vi "Setpoint.vi"(8 "error in (no error)":errorcluster, 10 "Setpoint [A]":dbl format="%.5f", 11 "PS Driver AMI4xx.lvlib:PS Driver AMI4xx.lvclass in":refnum<class "PS Driver AMI4xx.lvclass">) -> (0 "error out":errorcluster, 2 "Setpoint out (A)":dbl, 3 "PS Driver AMI4xx.lvlib:PS Driver AMI4xx.lvclass out":refnum<class "PS Driver AMI4xx.lvclass">)   [LabVIEW 2025, in "PS Driver.lvlib" / "PS Driver AMI4xx.lvclass"]
doc: "Author: Scott Hannahs <sth@magnet.fsu.edu>\n\nThis software is licensed for use under the “MIT License\"\nCopyright (c) 2025 Scott Hannahs, sth@sth@magnet.sthnet.net\n\nPermission is hereby granted, free of charge, to any person obtaining a copy of this software and associated documentation files (the \"Software\"), to deal in the Software without restriction, including without limitation the rights to use, copy, modify, merge, publish, distribute, sublicense, and/or sell copies of the Software, and to permit persons to whom the Software is furnished to do so, subject to the following conditions: The above copyright notice and this permission notice shall be included in all copies or substantial portions of the Software.\n\nTHE SOFTWARE IS PROVIDED \"AS IS\", WITHOUT WARRANTY OF ANY KIND, EXPRESS OR IMPLIED, INCLUDING BUT NOT LIMITED TO THE WARRANTIES OF MERCHANTABILITY, FITNESS FOR A PARTICULAR PURPOSE AND NONINFRINGEMENT. IN NO EVENT SHALL THE AUTHORS OR COPYRIGHT HOLDERS BE LIABLE FOR ANY CLAIM, DAMAGES OR OTHER LIABILITY, WHETHER IN AN ACTION OF CONTRACT, TORT OR OTHERWISE, ARISING FROM, OUT OF OR IN CONNECTION WITH THE SOFTWARE OR THE USE OR OTHER DEALINGS IN THE SOFTWARE."
uses:
  PS Driver AMI4xx.lvclass
  PS Driver with Persistence.lvclass
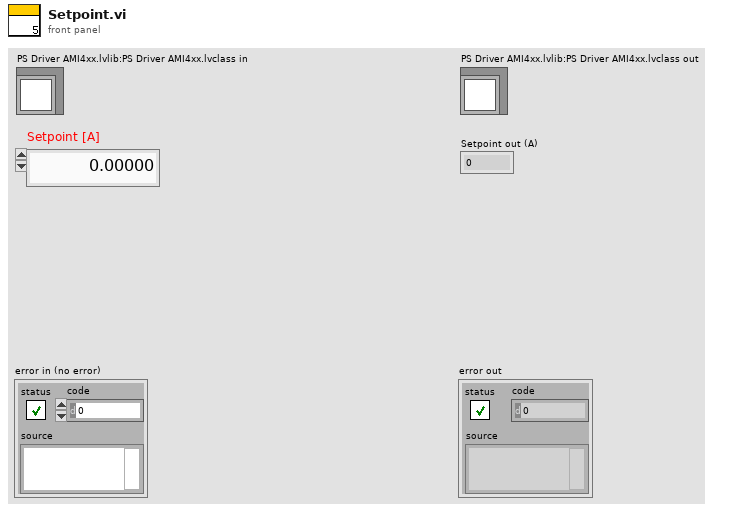
[diagram p1: front panel]
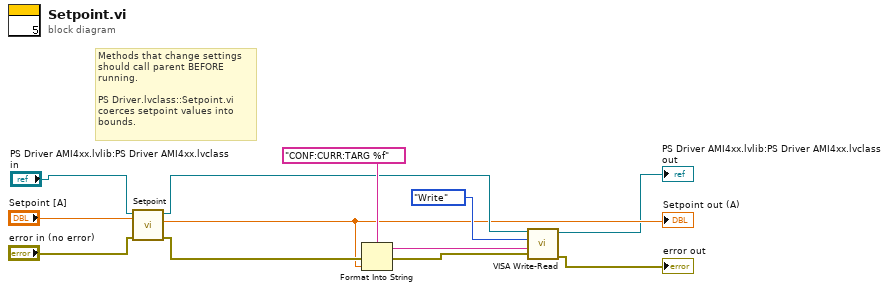
[diagram p0: block diagram]
diagram:
  # "Methods that change settings\nshould call parent BEFORE\nrunning.\n\nPS Driver.lvclass::Setpoint.vi \ncoerces setpoint values into\nbounds."
  n1 = call-parent "Setpoint.vi"("error in (no error)"="error in (no error)", "Setpoint [A]"="Setpoint [A]", "PS Driver.lvlib:PS Driver.lvclass in"="PS Driver AMI4xx.lvlib:PS Driver AMI4xx.lvclass in") -> ("error out"=w5:errorcluster, "Setpoint out (A)"=w2:dbl, "PS Driver.lvlib:PS Driver.lvclass out"=w7:refnum<class "PS Driver AMI4xx.lvclass">)  [unwired: 6 in]
  "Setpoint out (A)" <- w2
  n2 = Format Into String(format string="CONF:CURR:TARG %f" ("Command String"), error in=w5, w2) -> (resulting string=w10:string, error out=w4:errorcluster)  [unwired: 1 in]
  n3 = call "VISA Write-Read.vi"("error in (no error)"=w4, "Command String"=w10, "Action"=enum16{"Write", "Read", "Write & Read"}."Write", "PS Driver.lvlib:PS Driver AMI4xx.lvclass"=w7) -> ("error out"=→"error out":errorcluster, "PS Driver.lvlib:PS Driver AMI4xx.lvclass out"=→"PS Driver AMI4xx.lvlib:PS Driver AMI4xx.lvclass out":refnum<class "PS Driver AMI4xx.lvclass">)  [unwired: 4 in, 2 out]
